vi "Fetch Waveform Measurement.vi"(7 "Destination Channel (1: Channel 2)":u16(ring)=1 items=["Channel 1", "Channel 2", "Channel 3", "Channel 4", "Math", "D0", "D1", "D2", "D3", "D4", "D5", "D6", "D7", "D8", "D9", "D10", "D11", "D12", "D13", "D14", "D15", "Reference 1", "Reference 2", "Reference 3", "Reference 4", "Amplitude", "Frequency", "Phase"], 8 "error in (no error)":errorcluster, 9 "Measurement Function (0: Period)":i32(ring) items=["Period", "Frequency", "Delay", "Rise Time", "Fall Time", "Positive Duty Cycle", "Negative Duty Cycle", "Positive Pulse Width", "Negative Pulse Width", "Burst Width", "Phase", "Positive Overshoot", "Negative Overshoot", "Vpp", "Amplitude", "Voltage High", "Voltage Low", "Voltage Max", "Voltage Min", "Voltage Mean", "Voltage Mean (cycle)", "Voltage RMS", "Voltage RMS (cycle)", "Area", "Cycle Area", "Positive Edge Count", "Negative Edge Count", "Positive Pulse Count", "Negative Pulse Count", "Total Overshoot", "Histogram Hits", "Histogram Median", "Histogram Peak Hits", "Histogram Sigma 1", "Histogram Sigma 2", "Histogram Sigma 3", "Standard Deviation", "Waveform Count"], 10 "Channel (0: Channel 1)":u16(ring) items=["Channel 1", "Channel 2", "Channel 3", "Channel 4", "Math", "D0", "D1", "D2", "D3", "D4", "D5", "D6", "D7", "D8", "D9", "D10", "D11", "D12", "D13", "D14", "D15", "Reference 1", "Reference 2", "Reference 3", "Reference 4", "Amplitude", "Frequency", "Phase"], 11 "VISA resource name":refnum<visa-resource-name>) -> (0 "error out":errorcluster, 2 "Measurement Value":dbl, 3 "VISA resource name out":refnum<visa-resource-name>)   [LabVIEW 2017, in "Scope.lvlib" / "Tektronix DPO MSO 2000 4000 Series.lvlib"]
doc: "Initiates an acquisition on the channel that you specify in the <B>Channel</B> control. After the acquisition completes, the Fetch Waveform Measurement VI performs waveform measurement on the channel you specify and returns a measurement value. You can specify a measurement type, such as rise time, frequency, and voltage peak-to-peak, with this VI. Use the Fetch Waveform Measurement VI separately for any other waveform measurement on a channel without initiating another acquisition."
uses:
  Tektronix DPO MSO 2000 4000 Series.lvlib
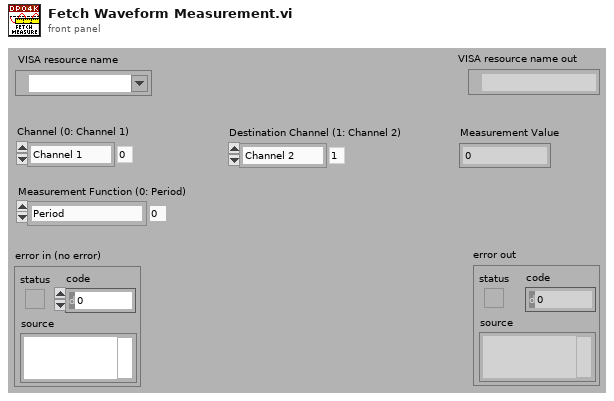
[diagram p1: front panel]
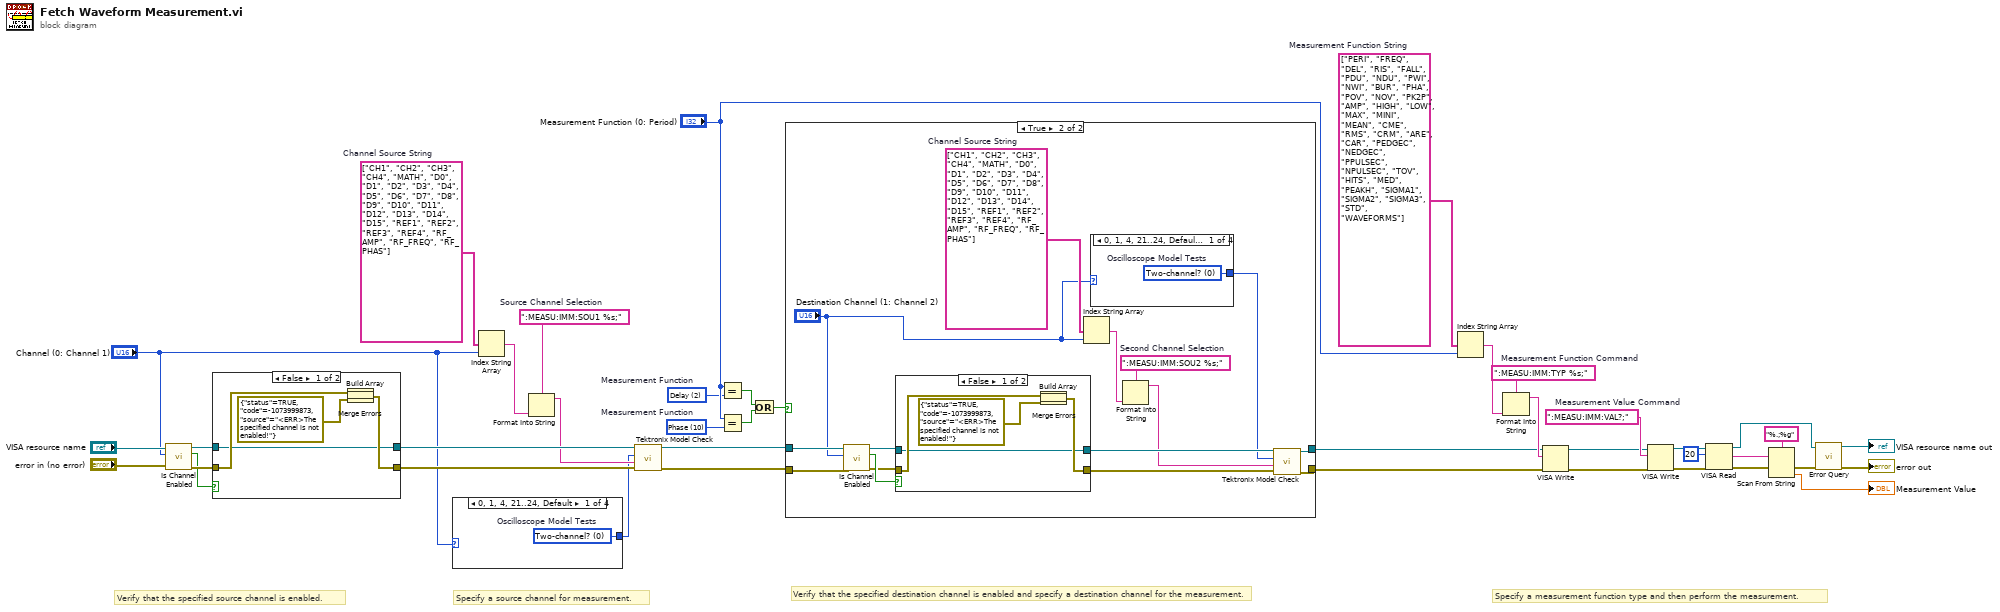
[diagram p0: block diagram]
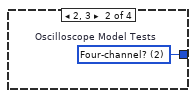
[diagram p2: hidden frame]
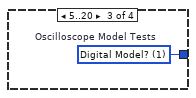
[diagram p3: hidden frame]
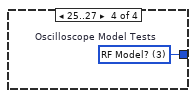
[diagram p4: hidden frame]
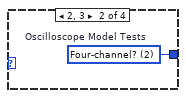
[diagram p7: hidden frame]
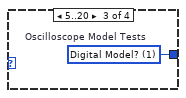
[diagram p8: hidden frame]
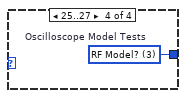
[diagram p9: hidden frame]
diagram:
  w2 = 10 items=["Period", "Frequency", "Delay", "Rise Time", "Fall Time", "Positive Duty Cycle", "Negative Duty Cycle", "Positive Pulse Width", "Negative Pulse Width", "Burst Width", "Phase", "Positive Overshoot", "Negative Overshoot", "Vpp", "Amplitude", "Voltage High", "Voltage Low", "Voltage Max", "Voltage Min", "Voltage Mean", "Voltage Mean (cycle)", "Voltage RMS", "Voltage RMS (cycle)", "Area", "Cycle Area", "Positive Edge Count", "Negative Edge Count", "Positive Pulse Count", "Negative Pulse Count", "Total Overshoot"]  # Measurement Function
  w3 = 2 items=["Period", "Frequency", "Delay", "Rise Time", "Fall Time", "Positive Duty Cycle", "Negative Duty Cycle", "Positive Pulse Width", "Negative Pulse Width", "Burst Width", "Phase", "Positive Overshoot", "Negative Overshoot", "Vpp", "Amplitude", "Voltage High", "Voltage Low", "Voltage Max", "Voltage Min", "Voltage Mean", "Voltage Mean (cycle)", "Voltage RMS", "Voltage RMS (cycle)", "Area", "Cycle Area", "Positive Edge Count", "Negative Edge Count", "Positive Pulse Count", "Negative Pulse Count", "Total Overshoot"]  # Measurement Function
  w15 = ":MEASU:IMM:SOU1 %s;"  # Source Channel Selection
  w14 = string[] ["CH1", "CH2", "CH3", "CH4", "MATH", "D0", "D1", "D2", "D3", "D4", "D5", "D6", "D7", "D8", "D9", "D10", "D11", "D12", "D13", "D14", "D15", "REF1", "REF2", "REF3", "REF4", "RF_AMP", "RF_FREQ", "RF_PHAS"]  # Channel Source String
  w32 = ":MEASU:IMM:VAL?;"  # Measurement Value Command
  w40 = ":MEASU:IMM:TYP %s;"  # Measurement Function Command
  w41 = string[] ["PERI", "FREQ", "DEL", "RIS", "FALL", "PDU", "NDU", "PWI", "NWI", "BUR", "PHA", "POV", "NOV", "PK2P", "AMP", "HIGH", "LOW", "MAX", "MINI", "MEAN", "CME", "RMS", "CRM", "ARE", "CAR", "PEDGEC", "NEDGEC", "PPULSEC", "NPULSEC", "TOV", "HITS", "MED", "PEAKH", "SIGMA1", "SIGMA2", "SIGMA3", "STD", "WAVEFORMS"]  # Measurement Function String
  # "Specify a measurement function type and then perform the measurement."
  # "Verify that the specified destination channel is enabled and specify a destination channel for the measurement."
  # "Specify a source channel for measurement."
  # "Verify that the specified source channel is enabled."
  n1 = call "Is Channel Enabled.vi"("error in (no error)"="error in (no error)", "Channel (0: Channel 1)"="Channel (0: Channel 1)", "VISA resource name"="VISA resource name") -> ("error out"=w18:errorcluster, "Enabled"=w17:bool, "VISA resource name out"=w19:refnum<visa-resource-name>)  [unwired: 6 in]
  n2 = case shown="False" w17 {
    tunnel: w19 -> [w43 w48]
    tunnel: w18 -> [w45 w47]
    tunnel: [w43 w48] -> w10
    tunnel: [w44 w47] -> w9
    frame False {
      n3 = Build Array(w45, errorcluster {"status"=TRUE, "code"=-1073999873, "source"="<ERR>The specified channel is not enabled!"} ("error out")) -> (w42:errorcluster[])
      n4 = Merge Errors(w42) -> (w44:errorcluster)
    }
    frame True {
    }
  }
  n5 = case shown="0, 1, 4, 21..24, Default" "Channel (0: Channel 1)" {
    tunnel: [w49 w50 w51 w52] -> w5
    frame 0, 1, 4, 21..24, Default {
      w49 = u16 0 items=["Two-channel?", "Digital Model?", "Four-channel?", "RF Model?"]  # Oscilloscope Model Tests
    }
    frame 2, 3 {
      w50 = u16 2 items=["Two-channel?", "Digital Model?", "Four-channel?", "RF Model?"]  # Oscilloscope Model Tests
    }
    frame 5..20 {
      w51 = u16 1 items=["Two-channel?", "Digital Model?", "Four-channel?", "RF Model?"]  # Oscilloscope Model Tests
    }
    frame 25..27 {
      w52 = u16 3 items=["Two-channel?", "Digital Model?", "Four-channel?", "RF Model?"]  # Oscilloscope Model Tests
    }
  }
  n6 = Index String Array(1:"Channel (0: Channel 1)", 2:w14) -> (0:w16:string)  [unwired: 1 in]
  n7 = Format Into String(format string=w15, w16) -> (resulting string=w8:string)  [unwired: 2 in, 1 out]
  n8 = call "Tektronix Model Check.vi"("error in (no error)"=w9, "Command String"=w8, "Oscilloscope Model Tests (3: RF Model?)"=w5, "VISA resource name"=w10) -> ("error out"=w6:errorcluster, "VISA resource name out"=w7:refnum<visa-resource-name>)  [unwired: 6 in]
  n9 = Equal?(x="Measurement Function (0: Period)", y=w3) -> (x = y?=w38:bool)
  n10 = Equal?(x="Measurement Function (0: Period)", y=w2) -> (x = y?=w37:bool)
  n11 = Or(x=w38, y=w37) -> (x .or. y?=w36:bool)
  n12 = case shown="True" w36 {
    tunnel: w7 -> [w54 w67]
    tunnel: w6 -> [w53 w66]
    tunnel: [w54 w58] -> w34
    tunnel: [w53 w57] -> w33
    frame False {
    }
    frame True {
      w62 = string[] ["CH1", "CH2", "CH3", "CH4", "MATH", "D0", "D1", "D2", "D3", "D4", "D5", "D6", "D7", "D8", "D9", "D10", "D11", "D12", "D13", "D14", "D15", "REF1", "REF2", "REF3", "REF4", "RF_AMP", "RF_FREQ", "RF_PHAS"]  # Channel Source String
      w68 = ":MEASU:IMM:SOU2 %s;"  # Second Channel Selection
      n13 = call "Is Channel Enabled.vi"("error in (no error)"=w66, "Channel (0: Channel 1)"="Destination Channel (1: Channel 2)", "VISA resource name"=w67) -> ("error out"=w63:errorcluster, "Enabled"=w65:bool, "VISA resource name out"=w64:refnum<visa-resource-name>)  [unwired: 6 in]
      n14 = case shown="False" w65 {
        tunnel: w64 -> [w75 w80]
        tunnel: w63 -> [w77 w79]
        tunnel: [w75 w80] -> w61
        tunnel: [w76 w79] -> w60
        frame False {
          n15 = Build Array(w77, errorcluster {"status"=TRUE, "code"=-1073999873, "source"="<ERR>The specified channel is not enabled!"} ("error out")) -> (w74:errorcluster[])
          n16 = Merge Errors(w74) -> (w76:errorcluster)
        }
        frame True {
        }
      }
      n17 = Index String Array(1:"Destination Channel (1: Channel 2)", 2:w62) -> (0:w69:string)  [unwired: 1 in]
      n18 = case shown="0, 1, 4, 21..24, Default" "Destination Channel (1: Channel 2)" {
        tunnel: [w70 w71 w72 w73] -> w55
        frame 0, 1, 4, 21..24, Default {
          w70 = u16 0 items=["Two-channel?", "Digital Model?", "Four-channel?", "RF Model?"]  # Oscilloscope Model Tests
        }
        frame 2, 3 {
          w71 = u16 2 items=["Two-channel?", "Digital Model?", "Four-channel?", "RF Model?"]  # Oscilloscope Model Tests
        }
        frame 5..20 {
          w72 = u16 1 items=["Two-channel?", "Digital Model?", "Four-channel?", "RF Model?"]  # Oscilloscope Model Tests
        }
        frame 25..27 {
          w73 = u16 3 items=["Two-channel?", "Digital Model?", "Four-channel?", "RF Model?"]  # Oscilloscope Model Tests
        }
      }
      n19 = Format Into String(format string=w68, w69) -> (resulting string=w59:string)  [unwired: 2 in, 1 out]
      n20 = call "Tektronix Model Check.vi"("error in (no error)"=w60, "Command String"=w59, "Oscilloscope Model Tests (3: RF Model?)"=w55, "VISA resource name"=w61) -> ("error out"=w57:errorcluster, "VISA resource name out"=w58:refnum<visa-resource-name>)  [unwired: 6 in]
    }
  }
  n21 = Index String Array(1:"Measurement Function (0: Period)", 2:w41) -> (0:w39:string)  [unwired: 1 in]
  n22 = Format Into String(format string=w40, w39) -> (resulting string=w35:string)  [unwired: 2 in, 1 out]
  n23 = VISA Write(VISA resource name=w34, write buffer=w35, error in (no error)=w33) -> (VISA resource name out=w25:refnum<visa-resource-name>, error out=w24:errorcluster)  [unwired: 1 out]
  n24 = VISA Write(VISA resource name=w25, write buffer=w32, error in (no error)=w24) -> (VISA resource name out=w31:refnum<visa-resource-name>, error out=w30:errorcluster)  [unwired: 1 out]
  n25 = VISA Read(VISA resource name=w31, byte count=u32 20, error in (no error)=w30) -> (VISA resource name out=w11:refnum<visa-resource-name>, read buffer=w28:string, error out=w13:errorcluster)  [unwired: 1 out]
  n26 = Scan From String(format string="%.;%g", input string=w28, error in=w13) -> (error out=w12:errorcluster, output 1=→"Measurement Value":dbl)  [unwired: 2 in, 2 out]
  n27 = call "Error Query.vi"("error in (no error)"=w12, "VISA resource name"=w11) -> ("error out"=→"error out":errorcluster, "VISA resource name out"=→"VISA resource name out":refnum<visa-resource-name>)  [unwired: 6 in, 2 out]
